vi "DirExists-NoThenCreate.vi"(2 "error in":errorcluster, 3 "path":path) -> (0 "error out":errorcluster, 1 "created path":path)   [LabVIEW 2011]
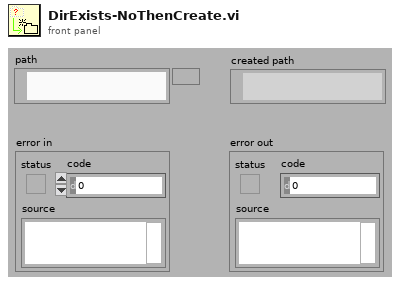
[diagram p1: front panel]
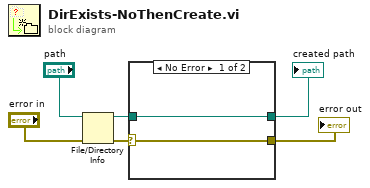
[diagram p0: block diagram]
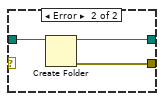
[diagram p2: hidden frame]
diagram:
  n1 = File/Directory Info(path="path", error in="error in") -> (path out=w5:path, error out=w6:errorcluster)  [unwired: 5 out]
  n2 = case shown="No Error" w6 {
    selector: w6 -> [w8 _]
    tunnel: w5 -> [w7 w11]
    tunnel: [w8 w10] -> w4
    tunnel: [w7 w9] -> w1
    frame No Error {
    }
    frame Error {
      n3 = Create Folder(path (use dialog)=w11) -> (created path=w9:path, error out=w10:errorcluster)  [unwired: 1 in, 2 out]
    }
  }
  "error out" <- w4
  "created path" <- w1
